vi "HEWH Header Length.vi"(7 "DBL?":bool, 8 "error in (no error)":errorcluster, 9 "Full Data String":string[][](array[string]), 11 "Full Data DBL":dbl[][](array[numeric])) -> (0 "error out":errorcluster, 1 "Full Data String":string[][](array[string]), 3 "Full Data DBL Out":dbl[][](array[numeric]), 4 "Header Length":i32)   [LabVIEW 2023]
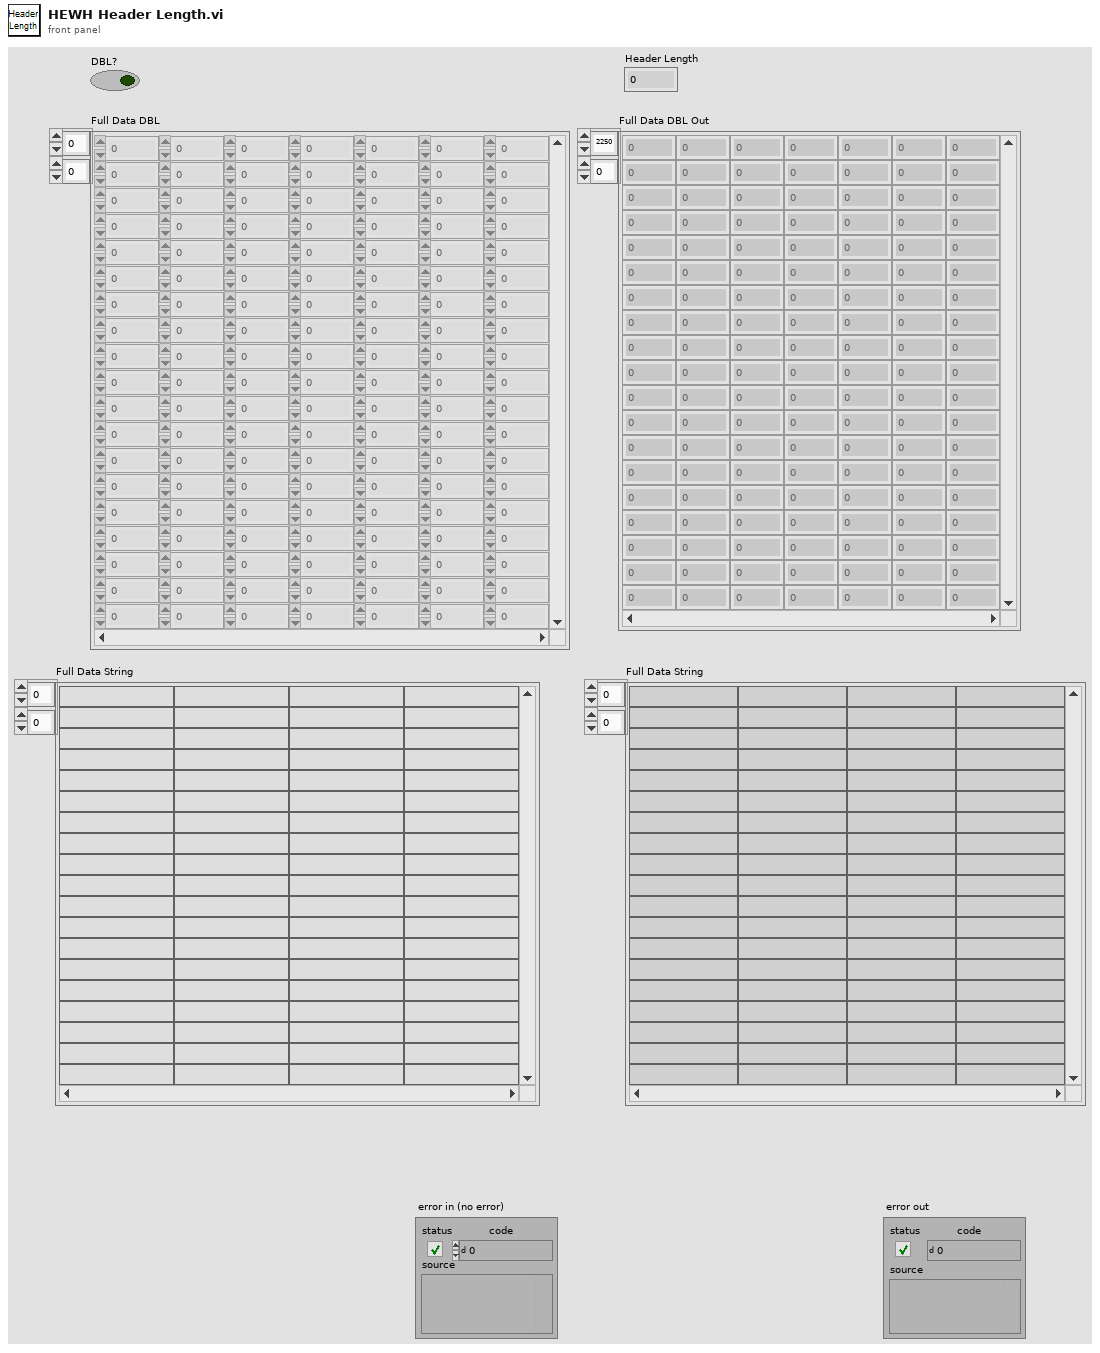
[diagram p1: front panel]
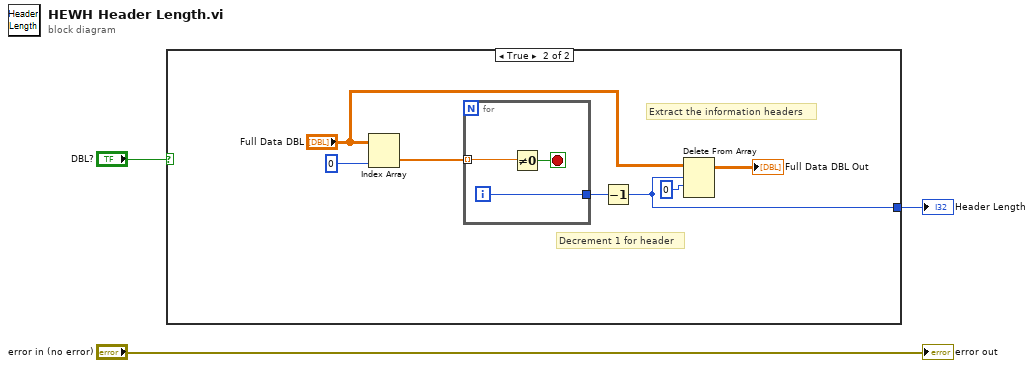
[diagram p0: block diagram]
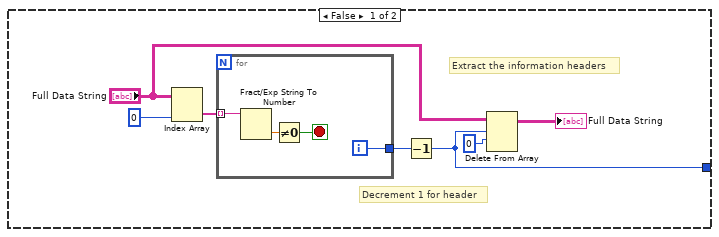
[diagram p2: hidden frame]
diagram:
  n1 = case shown="True" "DBL?" {
    tunnel: [w4 w17] -> w2
    frame False {
      # "Decrement 1 for header"
      # "Extract the information headers"
      n2 = Index Array(array="Full Data String", index (col)=0 ("disabled index (col)")) -> (element=w10:string[])  [unwired: 1 in]
      n3 = for {
        tunnel: w10 -> [w13] mode=indexing
        tunnel: [w11] -> w9
        i -> [w11]
        stop <- w14 stop-if-true
        n4 = Fract/Exp String To Number(string=w13) -> (number=w12:dbl)  [unwired: 3 in, 1 out]
        n5 = Not Equal To 0?(x=w12) -> (x != 0?=w14:bool)
      }
      n6 = Decrement(x=w9) -> (x-1=w4:i32)
      n7 = Delete From Array(array="Full Data String", length=w4, index (row)=0 ("index")) -> (array with subset deleted=→"Full Data String":string[][])  [unwired: 1 in, 1 out]
    }
    frame True {
      # "Decrement 1 for header"
      # "Extract the information headers"
      n8 = Index Array(array="Full Data DBL", index (col)=0 ("disabled index (col)")) -> (element=w19:dbl[])  [unwired: 1 in]
      n9 = for {
        tunnel: w19 -> [w24] mode=indexing
        tunnel: [w22] -> w18
        i -> [w22]
        stop <- w23 stop-if-true
        n10 = Not Equal To 0?(x=w24) -> (x != 0?=w23:bool)
      }
      n11 = Decrement(x=w18) -> (x-1=w17:i32)
      n12 = Delete From Array(array="Full Data DBL", length=w17, index (row)=0 ("index")) -> (array with subset deleted=→"Full Data DBL Out":dbl[][])  [unwired: 1 in, 1 out]
    }
  }
  "Header Length" <- w2
  "error out" <- "error in (no error)"
